vi "波形图表的构成.vi"() -> ()   [LabVIEW 2012]
panel:
  in  "停止":bool
  out "波形图表":T1(graph)
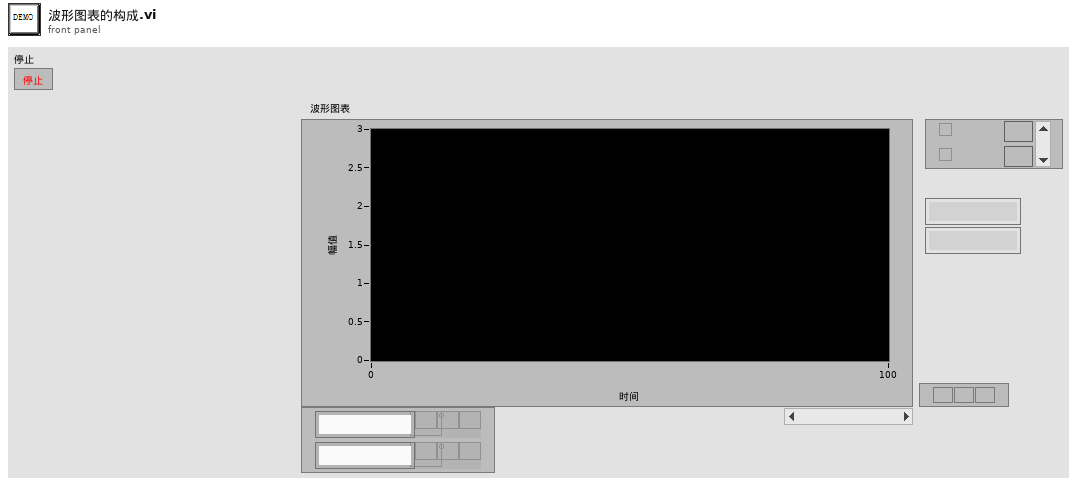
[diagram p1: front panel]
types:
  T1 = cluster{"number: 0 to 1":dbl, "number: 0 to 1":dbl}[]
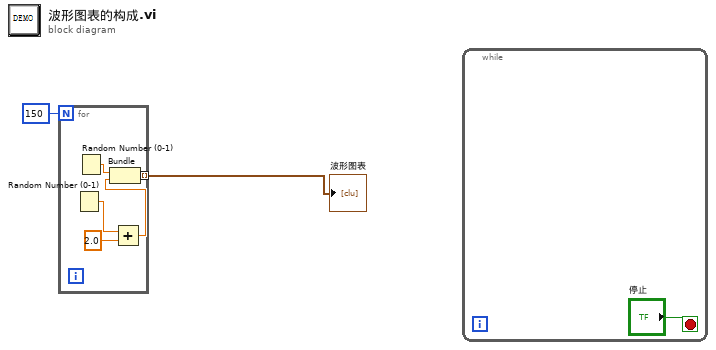
[diagram p0: block diagram]
diagram:
  n1 = for {
    N: 150 -> [_]
    tunnel: [w6] -> w1 mode=indexing
    n2 = Random Number (0-1)() -> (number: 0 to 1=w5:dbl)
    n3 = Random Number (0-1)() -> (number: 0 to 1=w7:dbl)
    n4 = Add(x=w5, y=2.0) -> (x+y=w3:dbl)
    n5 = Bundle("number: 0 to 1"=w7, w3) -> (w6:cluster{"number: 0 to 1":dbl, dbl})  [unwired: 1 in]
  }
  "波形图表" <- w1
  n6 = while {
    stop <- "停止" stop-if-true
  }
